vi "Main-Auto_Lite.vi"() -> ()   [LabVIEW 2019]
uses:
  <vilib>/myRIO/Instrument Drivers/Onboard IO/DIO/typedefs/DIO Reference.ctl
  <vilib>/myRIO/Common/Instrument Driver Framework/Utilities/typedefs/myRIO Generic Hardware Reference.ctl
  <vilib>/myRIO/Common/Instrument Driver Framework/Utilities/typedefs/Hardware Version Enum.ctl
  <vilib>/myRIO/Common/Instrument Driver Framework/Utilities/typedefs/myRIO v1.0 Reference.ctl
  <vilib>/myRIO/Common/Instrument Driver Framework/Utilities/typedefs/Generic FPGA Reference.ctl
  <vilib>/myRIO/Common/Instrument Driver Framework/myRIO v1.0/DIO/typedefs/DIO Channels List.ctl
  <vilib>/myRIO/Common/Instrument Driver Framework/myRIO v1.0/DIO/typedefs/DIO Channels Enum.ctl
  <vilib>/userDefined/High Color/nirio_resource_hc.ctl
  <vilib>/Platform/TimedLoop/XDataNode/timing_clust.ctl
  <vilib>/Platform/TimedLoop/XDataNode/nitl_modes.ctl
  <vilib>/Platform/TimedLoop/XDataNode/wakeup.ctl
  <vilib>/myRIO/Common/Instrument Driver Framework/Utilities/vis/Is FPGA Ref Available.vi
  <vilib>/myRIO/Common/Instrument Driver Framework/myRIO v1.0/DIO/vis/myRIO v1.1 Open DIO.vi
  <vilib>/myRIO/Instrument Drivers/Onboard IO/DIO/vis/Write.vi
  <vilib>/myRIO/Common/Instrument Driver Framework/Utilities/vis/Validate Channels.vi
  <vilib>/myRIO/Common/Instrument Driver Framework/myRIO v1.0/DIO/vis/myRIO v1.0 Reserve DIO.vi
  <vilib>/myRIO/Common/Instrument Driver Framework/myRIO v1.0/UART/vis/myRIO v1.0 Close UART.vi
  <vilib>/myRIO/Common/Instrument Driver Framework/myRIO v1.0/Resource Manager/vis/myRIO v1.0 Reserve Channel List.vi
  <vilib>/myRIO/Common/Instrument Driver Framework/myRIO v1.0/DIO/vis/myRIO v1.0 Build MUX Configuration DIO.vi
  <vilib>/myRIO/Common/Instrument Driver Framework/myRIO v1.0/Resource Manager/vis/myRIO v1.0 Reserve Channel.vi
  <vilib>/myRIO/Common/Instrument Driver Framework/myRIO v1.0/Resource Manager/vis/myRIO v1.0 Unreserve Channel.vi
  <vilib>/myRIO/Common/Instrument Driver Framework/myRIO v1.0/Resource Manager/vis/myRIO v1.0 Create Configuration List.vi
  <vilib>/myRIO/Common/Instrument Driver Framework/myRIO v1.0/Resource Manager/vis/myRIO v1.0 Build Mutex Name.vi
  <vilib>/Utility/VariantDataType/GetNumericInfo.vi
  <vilib>/Utility/error.llb/Error Cluster From Error Code.vi
  <vilib>/myRIO/Common/Instrument Driver Framework/myRIO v1.0/myRIO v1.1 Open.vi
  <vilib>/myRIO/Common/Instrument Driver Framework/Utilities/vis/IO Manager.vi
  <vilib>/myRIO/Common/Instrument Driver Framework/Utilities/vis/Configuration Manager.vi
  <vilib>/myRIO/Common/Instrument Driver Framework/myRIO v1.0/Resource Manager/vis/myRIO v1.0 Configure IO.vi
  <vilib>/myRIO/Common/Instrument Driver Framework/myRIO v1.0/myRIO v1.0 Close.vi
  <vilib>/myRIO/Common/Instrument Driver Framework/myRIO v1.0/DIO/vis/myRIO v1.0 Write DIO.vi
  Sub VI/Variable/Go-Home.vi
  Sub VI/Variable/Lock-PID.vi
  <vilib>/myRIO/Common/Instrument Driver Framework/Utilities/vis/FPGA Ref Manager.vi
  <vilib>/myRIO/Common/Instrument Driver Framework/myRIO v1.0/myRIO v1.0 Reset FPGA.vi
  <vilib>/myRIO/Common/Instrument Driver Framework/myRIO v1.0/IRQ/vis/myRIO v1.0 IRQ Info FGV.vi
  <vilib>/myRIO/Common/Instrument Driver Framework/myRIO v1.0/IRQ/vis/myRIO v1.0 Timer IRQ Info FGV.vi
  <vilib>/myRIO/Common/Instrument Driver Framework/myRIO v1.0/IRQ/vis/myRIO v1.0 ISR Agent.vi
  <vilib>/myRIO/Instrument Drivers/Utilities/vis/Reset Index.vi
  <vilib>/myRIO/Common/Instrument Driver Framework/myRIO v1.0/Resource Manager/vis/myRIO v1.0 Block Write Resource Manager.vi
  <vilib>/myRIO/Express VI/Onboard Devices/LED/LED Express VI.xnode
  <vilib>/myRIO/Instrument Drivers/Onboard IO/DIO/vis/myRIO DIO Open.xnode
  <vilib>/platform/TimedLoop/XDataNode/XDataNode.xnode
  <vilib>/myRIO/Instrument Drivers/Utilities/Utilities.lvlib
  <vilib>/Platform/TimedLoop/XDataNode/XDNodeRunTimeDep.lvlib
  <vilib>/myRIO/Instrument Drivers/Onboard IO/DIO/DIO.lvlib
panel:
  out "總辨識機率":i32[](graph)
  out "第二次辨識機率":i32[](graph)
  out "第一次辨識機率":i32[](graph)
  out "辨識機率":dbl[](array[slide]) scale=0.0..10.0
  out "總辨識結果":string[](array[string])
  out "輸出顏色-位置":T1(array[cluster])
  out "當前動作":enum16{"辨識", "夾球+回橋"}(ring)
  in  "Stop":bool
  out "Error Out":errorcluster
  in  "Error In":errorcluster
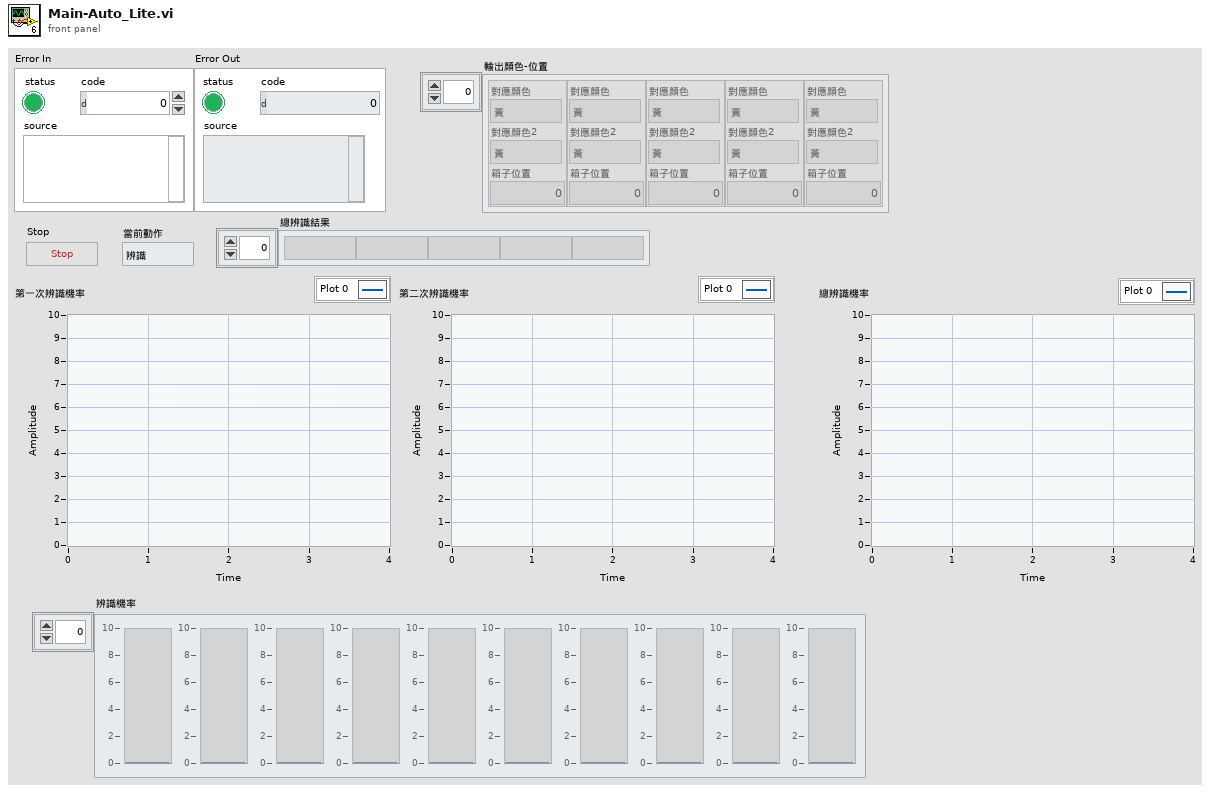
[diagram p1: front panel]
types:
  T1 = cluster{"對應顏色":enum16{"黃", "紅", "綠", "藍", "黑", "無"}, "對應顏色2":enum16{"黃", "紅", "綠", "藍", "黑", "無"}, "箱子位置":i32}[]
  T2 = enum16{"前", "後", "オ", "右", "無", "0", "1", "2", "3", "4", "5", "6", "7"}
  T3 = enum16{"第一次夾球", "第二次夾球", "第三次夾球", "第四次夾球", "第五次夾球"}
  T4 = enum16{"第一次夾球", "第二次夾球", "第三次夾球", "第四次夾球", "第五次夾球"}[]
  T5 = typedef "I2C.lvlib/I2C Reference.ctl" = cluster{"myRIO Reference":T6, "I2C Channels Enum":T10, "I2C Configuration":T11}
  T6 = typedef "myRIO Generic Hardware Reference.ctl" = cluster{"myRIO Model":T7, "myRIO Hardware Reference":T8}
  T7 = typedef "Hardware Version Enum.ctl" = enum16{"Unknown", "myRIO-1900", "myRIO-1950", "roboRIO", "NI ELVIS RIO CM", "ELVIS III"}
  T8 = typedef "myRIO v1.0 Reference.ctl" = cluster{"Generic FPGA Reference":T9, "Allow multiple opens":bool}
  T9 = typedef "Generic FPGA Reference.ctl" = refnum<k20>
  T10 = typedef "I2C Channels Enum.ctl" = enum16{"Not Connected", "A/I2C", "B/I2C", "I2C/I2C"}
  T11 = typedef "I2C.lvlib/I2C Configuration.ctl" = cluster{"I2C Transfer Rate":T12}
  T12 = typedef "I2C.lvlib/I2C Transfer Rate.ctl" = enum16{"Standard mode (100 kbps)", "Fast mode (400 kbps)"}
  T13 = cluster{"Array":i32[], "Array":i32[], "Array":i32[]}
  T14 = typedef "XDNodeRunTimeDep.lvlib/timing_clust.ctl" = cluster{"Expected End [f-1]":u64, "Actual End [f-1]":u64, "Finished Late? [f-1]":bool, "Expected End [i-1]":u64, "Actual End [i-1]":u64, "Finished Late? [i-1]":bool, "Expected Start [i]":u64, "Actual Start [i]":u64, "Expected Start [f]":u64, "Actual Start [f]":u64, "Source Name":string, "Structure Name":string, "Period":i64, "Deadline":i64, "Offset":i64, "Start":i64, "Priority":i32, "Timeout":i32, "Mode":T15, "Wakeup Reason":T16, "Error":errorcluster, "Source Type":string, "Secondary Source Type":string, "Global End Time":u64, "Global Start Time":u64, "Frame Duration":u64, "Iteration Duration":u64, "Assigned CPU":i32, "I/O Scan Engine Mode":u32}
  T15 = typedef "XDNodeRunTimeDep.lvlib/nitl_modes.ctl" = enum32{"No Change", "Process missed periods, maintain original phase", "Discard missed periods, maintain original phase", "Process missed periods, ignore original phase", "Discard missed periods, ignore original phase"}
  T16 = typedef "XDNodeRunTimeDep.lvlib/wakeup.ctl" = enum32{"Normal", "Aborted", "Asynchronous wakeup", "Timing source error", "Timed loop error", "Timeout"}
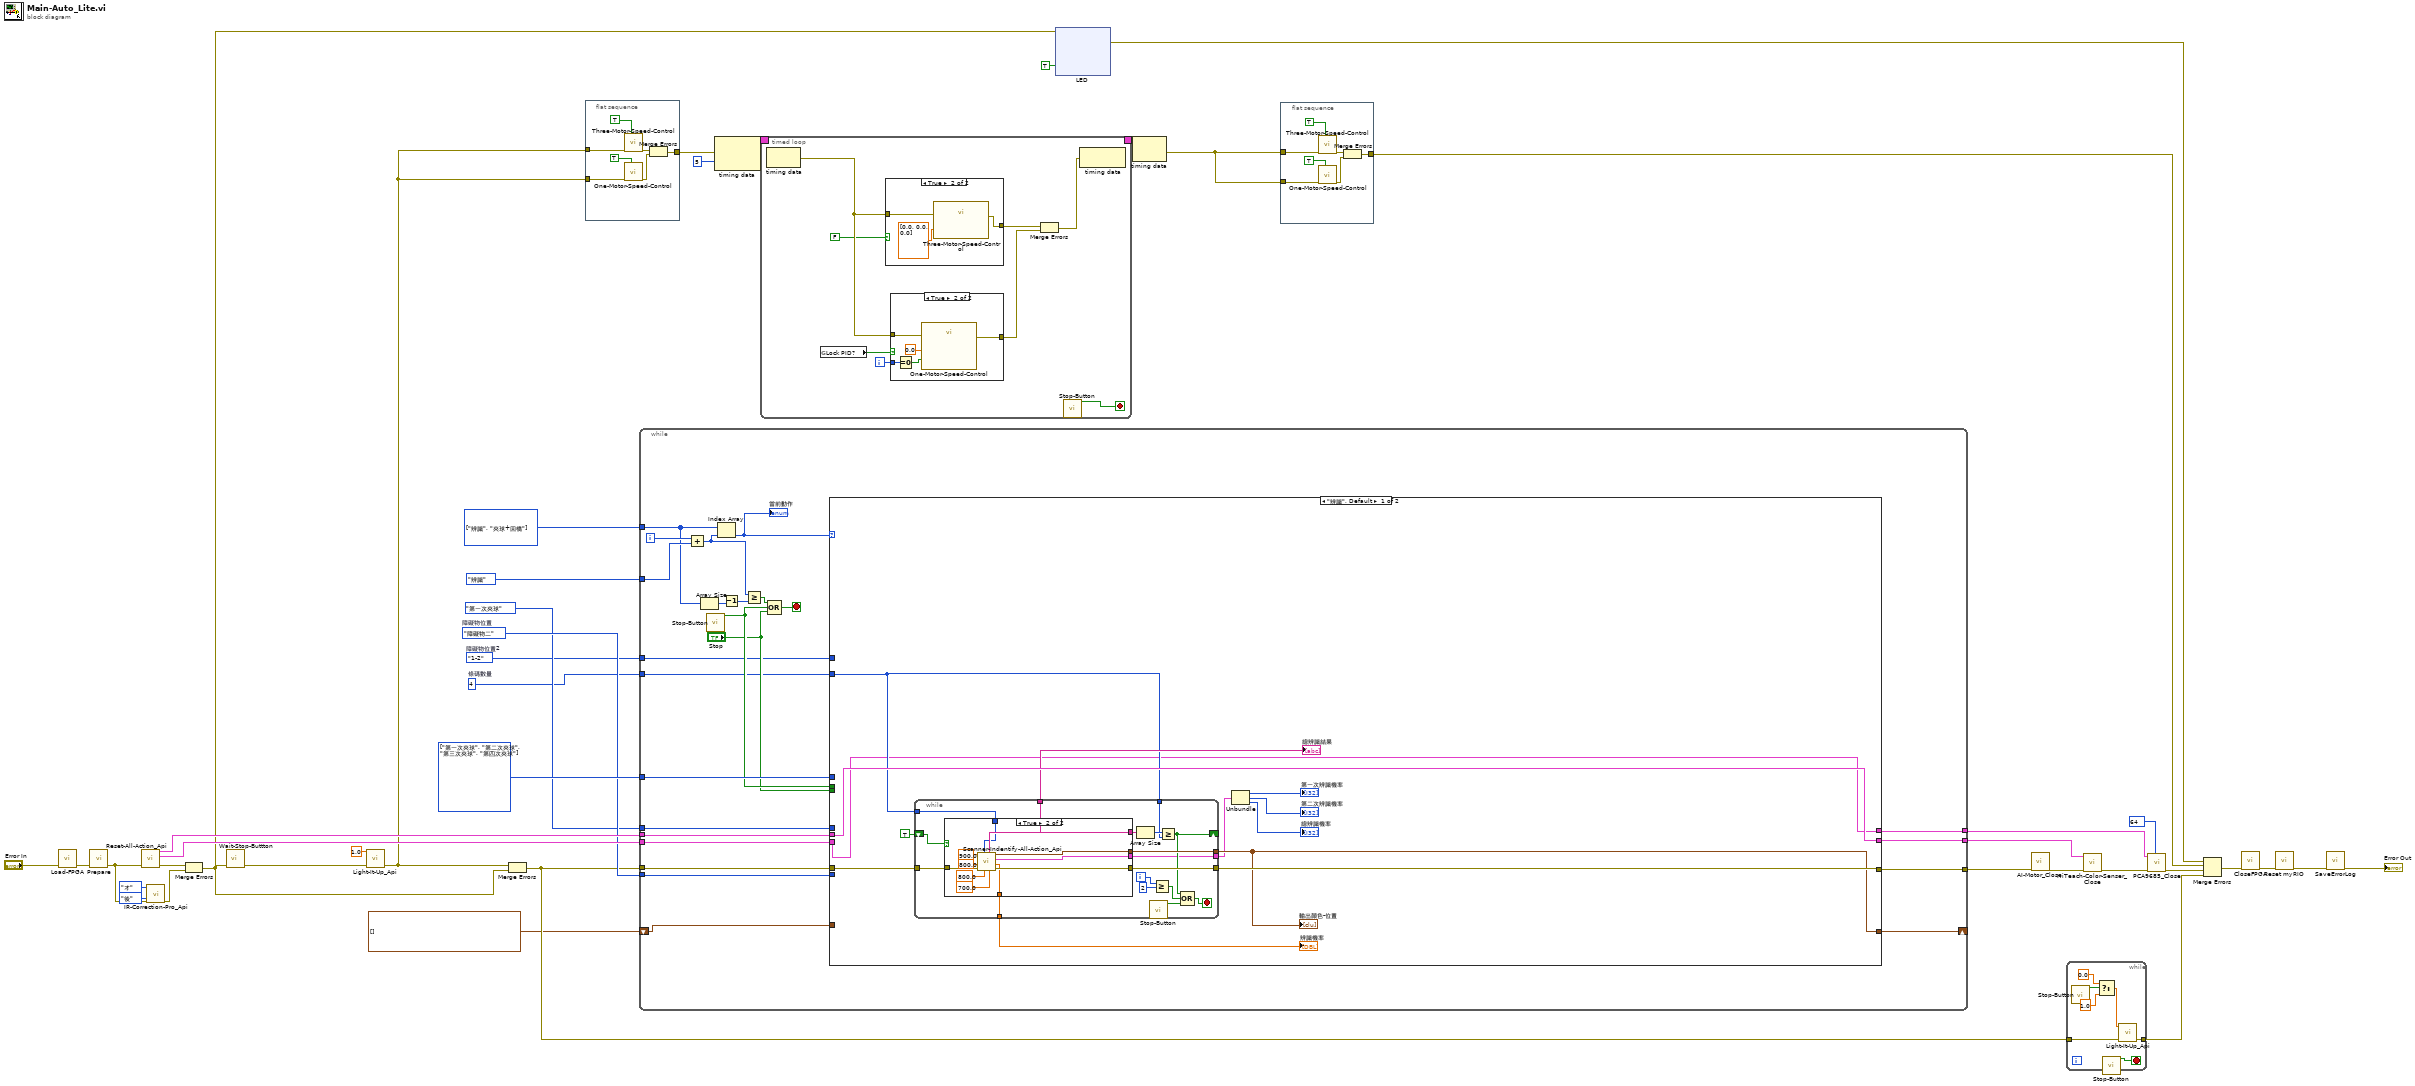
[diagram p0: block diagram]
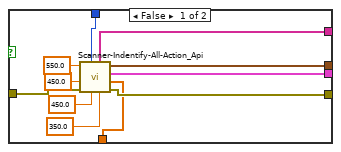
[diagram p2: hidden frame]
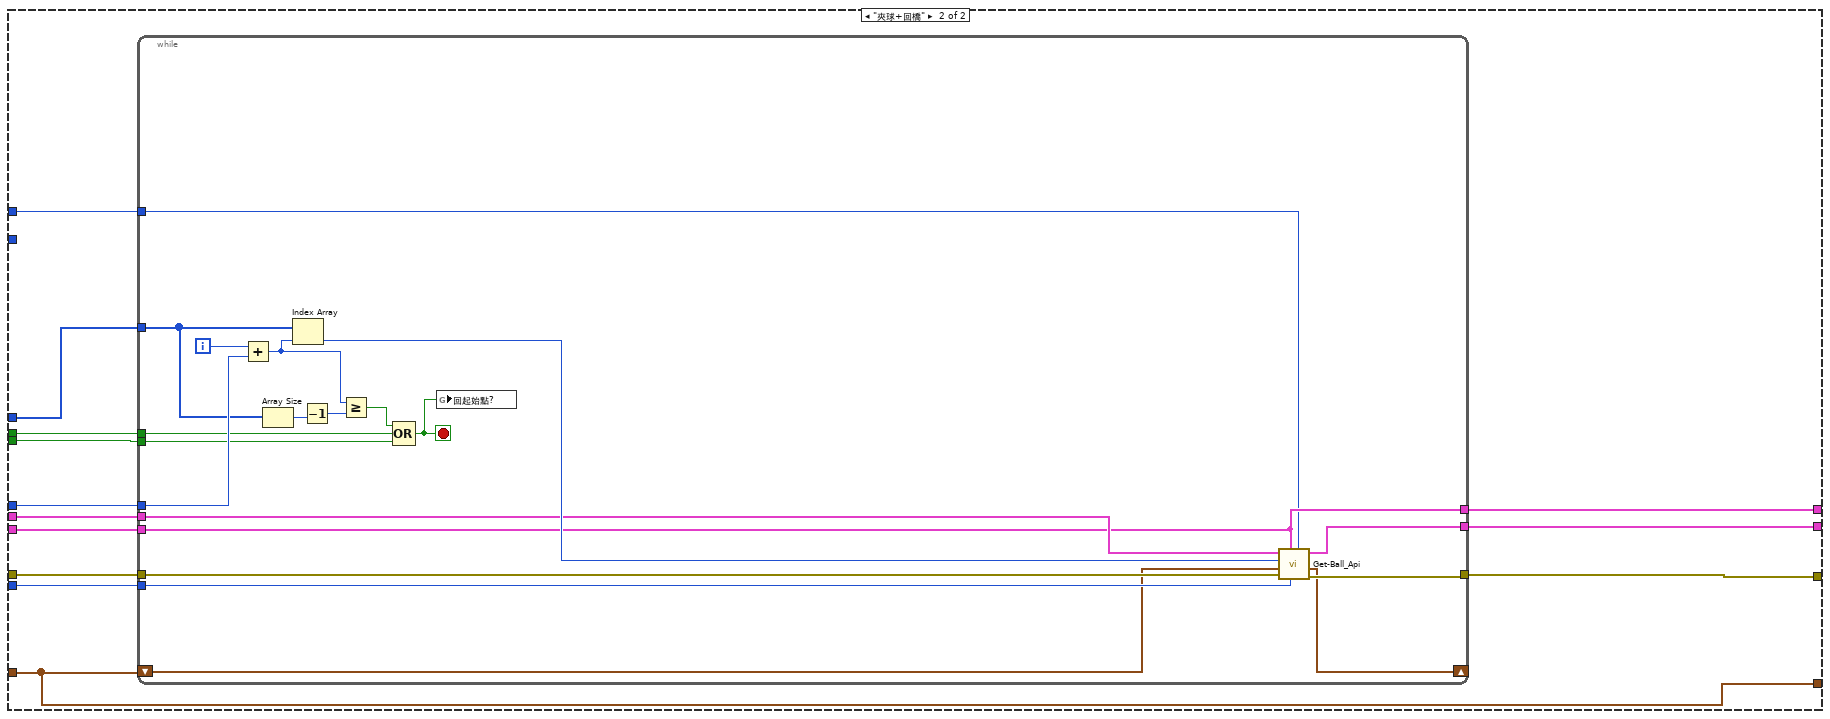
[diagram p3: hidden frame]
diagram:
  w11 = 4  # 條碼數量
  w13 = enum16{"1-1", "1-2", "2-1", "2-2"}."1-2"  # 障礙物位置2
  w25 = enum16{"障礙物一", "障礙物二"}."障礙物二"  # 障礙物位置
  w39 = T4 [enum."第一次夾球", enum."第二次夾球", enum."第三次夾球", enum."第四次夾球"] items=["第一次夾球", "第二次夾球", "第三次夾球", "第四次夾球", "第五次夾球"]
  w42 = enum16{"辨識", "夾球+回橋"}[] [enum."辨識", enum."夾球+回橋"] items=["辨識", "夾球+回橋"]
  n1 = call "Load-FPGA.vi"("Error In"="Error In") -> ("Error Out"=w8:errorcluster)  [unwired: 10 in]
  n2 = call "Prepare.vi"("Error In"=w8) -> ("Error Out"=w6:errorcluster)  [unwired: 10 in]
  n3 = call "Reset-All-Action_Api.vi"("Error In"=w6) -> ("Error Out"=w2:errorcluster, "I2C Ref Out"=w33:T5, "HiTechnicColorSensorV2 Ref Out"=w36:cluster{"I2C Ref Out":T5})  [unwired: 8 in]
  n4 = call "IR-Correction-Pro_Api.vi"("Error In"=w6, "副邊校正"=T2."後", "主編校正"=enum16{"前", "後", "オ", "右", "無"}."オ") -> ("Error Out"=w1:errorcluster)  [unwired: 8 in]
  n5 = Merge Errors(w2, w1) -> (w3:errorcluster)
  n6 = call "Wait-Stop-Buttton.vi"("Error In"=w3) -> ("Error Out"=w24:errorcluster)  [unwired: 10 in]
  n7 = call "Light-It-Up_Api.vi"("error in (no error)"=w24, "Duty Cycle"=1.0) -> ("error out"=w7:errorcluster)  [unwired: 9 in]
  n8 = Merge Errors(w7, w3) -> (w20:errorcluster)
  n9 = flat-sequence {
    tunnel: w7 -> [w49]
    tunnel: w7 -> [w48]
    tunnel: [w45] -> w26
    frame #0 {
      n10 = call "Three-Motor-Speed-Control.vi"("Reset"=TRUE, "Error In"=w49) -> ("Error Out"=w47:errorcluster)  [unwired: 9 in]
      n11 = call "One-Motor-Speed-Control.vi"("Reset"=TRUE, "Error In"=w48) -> ("Error Out"=w46:errorcluster)  [unwired: 9 in]
      n12 = Merge Errors(w47, w46) -> (w45:errorcluster)
    }
  }
  n13 = while {
    tunnel: w42 -> [w63]
    tunnel: enum16{"辨識", "夾球+回橋"}."辨識" -> [w73]
    tunnel: w20 -> [w72]
    tunnel: [w71] -> w12
    tunnel: T3."第一次夾球" ("夾球開始位置") -> [w68]
    tunnel: w39 -> [w62]
    shift-right: [w59] -> _
    shift-left: T1 [] ("輸出顏色-位置") -> [w58]
    tunnel: w36 -> [w56]
    tunnel: [w55] -> w35
    tunnel: w33 -> [w52]
    tunnel: [w54] -> w34
    tunnel: w25 -> [w53]
    tunnel: w13 -> [w51]
    tunnel: w11 -> [w50]
    i -> [w69]
    stop <- w70 stop-if-true
    n14 = Add(x=w69, y=w73) -> (x+y=w66:i32)
    n15 = Array Size(array=w63) -> (size(s)=w65:i32)
    n16 = call "Stop-Button.vi"() -> ("顯示按下?"=w61:bool)  [unwired: 10 in, 1 out]
    n17 = Index Array(array=w63, index=w66) -> (element=w57:enum16{"辨識", "夾球+回橋"})
    "當前動作" <- w57
    n18 = Decrement(x=w65) -> (x-1=w64:i32)
    n19 = Greater Or Equal?(x=w66, y=w64) -> (x >= y?=w67:bool)
    n20 = Compound Arithmetic op=OR(w67, w61, "Stop") -> (w70:bool)
    n21 = case shown="\"辨識\", Default" w57 {
      tunnel: w72 -> [w85 w137]
      tunnel: [w84 w136] -> w71
      tunnel: w68 -> [_ w135]
      tunnel: w62 -> [_ w134]
      tunnel: w61 -> [_ w133]
      tunnel: "Stop" -> [_ w132]
      tunnel: [w83 w131] -> w59
      tunnel: w58 -> [_ w131]
      tunnel: w56 -> [w86 w130]
      tunnel: [w86 w129] -> w55
      tunnel: w52 -> [w74 w128]
      tunnel: [w74 w127] -> w54
      tunnel: w53 -> [_ w126]
      tunnel: w51 -> [_ w125]
      tunnel: w50 -> [w80 _]
      frame "辨識", Default {
        n22 = while {
          tunnel: w85 -> [w102]
          tunnel: [w99] -> w84
          tunnel: [w98] -> w83
          tunnel: [w93] -> w82
          shift-right: [w92] -> _
          shift-left: TRUE -> [w91]
          tunnel: w80 -> [w90]
          tunnel: w80 -> [w89]
          tunnel: [w88] -> w79
          tunnel: [w87] -> w75
          i -> [w97]
          stop <- w100 stop-if-true
          n23 = case shown="True" w91 {
            tunnel: w102 -> [w111 w124]
            tunnel: [w112 w123] -> w99
            tunnel: [w113 w122] -> w98
            tunnel: [w105 w121] -> w93
            tunnel: w90 -> [w106 w118]
            tunnel: [w104 w115] -> w88
            tunnel: [w103 w114] -> w87
            frame False {
              n24 = call "Scanner-Indentify-All-Action_Api.vi"("加速度 (回頭)"=350.0, "最高速 (回頭)"=450.0, "Barcode數量"=w106, "Error In"=w111, "加速度"=450.0, "最高速"=550.0) -> ("error out"=w112:errorcluster, 1:"辨識機率"=w103:dbl[], 2:"辨識機率"=w104:T13, "輸出顏色-位置"=w113:T1, "總辨識結果"=w105:string[])  [unwired: 1 in]
            }
            frame True {
              n25 = call "Scanner-Indentify-All-Action_Api.vi"("加速度 (回頭)"=700.0, "最高速 (回頭)"=800.0, "Barcode數量"=w118, "Error In"=w124, "加速度"=800.0, "最高速"=900.0) -> ("error out"=w123:errorcluster, 1:"辨識機率"=w114:dbl[], 2:"辨識機率"=w115:T13, "輸出顏色-位置"=w122:T1, "總辨識結果"=w121:string[])  [unwired: 1 in]
            }
          }
          n26 = Array Size(array=w93) -> (size(s)=w101:i32)
          n27 = call "Stop-Button.vi"() -> ("顯示按下?"=w94:bool)  [unwired: 10 in, 1 out]
          n28 = Greater Or Equal?(x=w97, y=2) -> (x >= y?=w95:bool)
          n29 = Greater Or Equal?(x=w101, y=w89) -> (x >= y?=w92:bool)
          n30 = Compound Arithmetic op=OR(w92, w95, w94) -> (w100:bool)
        }
        "輸出顏色-位置" <- w83
        "總辨識結果" <- w82
        "辨識機率" <- w75
        n31 = Unbundle(w79) -> ("Array"=→"第一次辨識機率":i32[], "Array"=→"第二次辨識機率":i32[], "Array"=→"總辨識機率":i32[])
      }
      frame "夾球+回橋" {
        n32 = while {
          tunnel: w135 -> [w151]
          tunnel: w134 -> [w150]
          tunnel: w133 -> [w149]
          tunnel: w132 -> [w148]
          tunnel: w130 -> [w146]
          tunnel: [w145] -> w129
          tunnel: w128 -> [w144]
          tunnel: w137 -> [w157]
          tunnel: [w139] -> w136
          tunnel: [w144] -> w127
          tunnel: w126 -> [w143]
          tunnel: w125 -> [w141]
          shift-right: [w138] -> _
          shift-left: w131 -> [w140]
          i -> [w152]
          stop <- w142 stop-if-true
          n33 = Add(x=w152, y=w151) -> (x+y=w156:i32)
          n34 = Array Size(array=w150) -> (size(s)=w155:i32)
          n35 = Index Array(array=w150, index=w156) -> (element=w147:T3)
          n36 = Decrement(x=w155) -> (x-1=w154:i32)
          n37 = Greater Or Equal?(x=w156, y=w154) -> (x >= y?=w153:bool)
          n38 = Compound Arithmetic op=OR(w153, w149, w148) -> (w142:bool)
          n39 = global write "Go-Home.vi" "回起始點?"(w142) -> ()
          n40 = call "Get-Ball_Api.vi"("障礙物位置2"=w141, "障礙物位置"=w143, "I2C Ref In"=w144, "Error In"=w157, "輸出顏色-位置"=w140, "夾球開始位置"=w147, "HiTechnicColorSensorV2 Ref"=w146) -> ("Error Out"=w139:errorcluster, "輸出顏色-位置"=w138:T1, "HiTechnicColorSensorV2 Ref Out"=w145:cluster{"I2C Ref Out":T5})  [unwired: 2 in]
        }
      }
    }
  }
  n41 = node-c288(w26, i64 5 ("Period")) -> (w31:T14)
  n42 = timed-loop {
    timing: w31 -> [_]
    timing-out: [_] -> w30
    i -> [w158]
    stop <- w165 stop-if-true
    n43 = node-c288() -> (w164:errorcluster)  [unwired: 1 in]
    n44 = global read "Lock-PID.vi" "Lock PID?"() -> (w159:bool)
    n45 = case shown="True" FALSE {
      tunnel: w164 -> [w166 w167]
      tunnel: [w166 w168] -> w161
      frame False {
      }
      frame True {
        n46 = call "Three-Motor-Speed-Control.vi"("Error In"=w167, "速度(秒/度)"=dbl[] [0.0, 0.0, 0.0]) -> ("Error Out"=w168:errorcluster)  [unwired: 9 in]
      }
    }
    n47 = case shown="True" w159 {
      tunnel: w164 -> [w170 w174]
      tunnel: [w170 w173] -> w162
      tunnel: w158 -> [_ w172]
      frame False {
      }
      frame True {
        n48 = Equal To 0?(x=w172) -> (x = 0?=w171:bool)
        n49 = call "One-Motor-Speed-Control.vi"("Reset"=w171, "Error In"=w174, "速度(秒/度)"=0.0) -> ("Error Out"=w173:errorcluster)  [unwired: 8 in]
      }
    }
    n50 = Merge Errors(w161, w162) -> (w163:errorcluster)
    n51 = call "Stop-Button.vi"() -> ("顯示按下?"=w165:bool)  [unwired: 10 in, 1 out]
    n52 = node-c288(w163) -> ()  [unwired: 1 out]
  }
  n53 = xnode "LED"("LED1"=TRUE, "error in (no error)"=w3) -> ("error out"=w18:errorcluster)
  n54 = node-c288(w30) -> (w27:errorcluster)
  n55 = flat-sequence {
    tunnel: w27 -> [w187]
    tunnel: w27 -> [w186]
    tunnel: [w183] -> w19
    frame #0 {
      n56 = call "Three-Motor-Speed-Control.vi"("Reset"=TRUE, "Error In"=w187) -> ("Error Out"=w185:errorcluster)  [unwired: 9 in]
      n57 = call "One-Motor-Speed-Control.vi"("Reset"=TRUE, "Error In"=w186) -> ("Error Out"=w184:errorcluster)  [unwired: 9 in]
      n58 = Merge Errors(w185, w184) -> (w183:errorcluster)
    }
  }
  n59 = call "AI-Motor_Close.vi"("Error In"=w12) -> ("Error Out"=w32:errorcluster)  [unwired: 10 in]
  n60 = while {
    tunnel: w20 -> [w189]
    tunnel: [w194] -> w22
    stop <- w188 stop-if-true
    n61 = call "Stop-Button.vi"() -> ("顯示按下?"=w192:bool)  [unwired: 10 in, 1 out]
    n62 = Select(t=0.0, s=w192, f=1.0) -> (s? t:f=w193:dbl)
    n63 = call "Stop-Button.vi"() -> ("顯示按下?"=w188:bool)  [unwired: 10 in, 1 out]
    n64 = call "Light-It-Up_Api.vi"("error in (no error)"=w189, "Duty Cycle"=w193) -> ("error out"=w194:errorcluster)  [unwired: 9 in]
  }
  n65 = call "HiTeach-Color-Senser_Close.vi"("Error In"=w32, "HiTechnicColorSensorV2 Ref"=w35) -> ("Error Out"=w14:errorcluster)  [unwired: 9 in]
  n66 = call "PCA9685_Close.vi"("驅動板位址(0x40)"=u8 64, "Error In"=w14, "I2C Ref In"=w34) -> ("Error Out"=w28:errorcluster)  [unwired: 8 in]
  n67 = Merge Errors(w18, w19, w28, w22) -> (w21:errorcluster)
  n68 = call "CloseFPGA.vi"("Error In"=w21) -> ("Error Out"=w40:errorcluster)  [unwired: 10 in]
  n69 = call <vilib>:"Reset myRIO.vi"("error in (no error)"=w40) -> ("error out"=w10:errorcluster)  [unwired: 10 in]
  n70 = call "SaveErrorLog.vi"("Error In"=w10) -> ("error out"=→"Error Out":errorcluster)  [unwired: 10 in]
